vi "Create Log video.vi"(8 "error in (no error)":errorcluster, 11 "Acceleration Exceeded Log Folder":path=path "c:/logfiles") -> (0 "error out":errorcluster, 2 "AVI Refnum":T2)   [LabVIEW 2017]
uses:
  <vilib>/vision/Avi.llb/IMAQ AVI2 Refnum.ctl
  <vilib>/vision/Image Controls.llb/IMAQ Image.ctl
  <vilib>/userdefined/High Color/IMAQdx.ctl
  <vilib>/vision/driver/NI_Vision_Acquisition_Software.lvlib
panel:
  out "New Image":T1
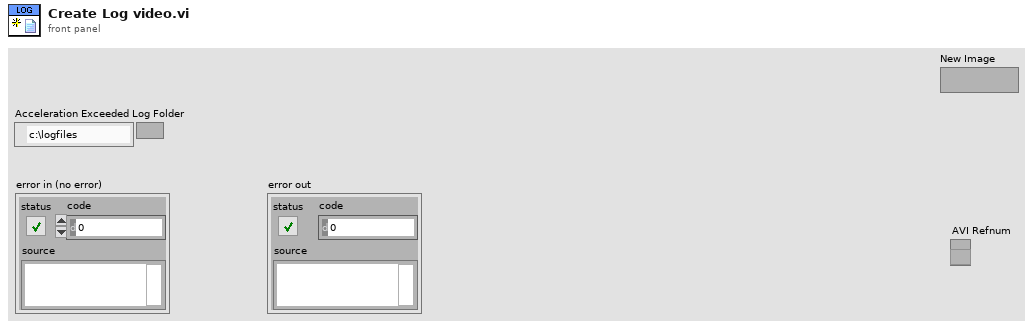
[diagram p1: front panel]
types:
  T1 = typedef "IMAQ Image.ctl" = refnum<image>
  T2 = typedef "IMAQ AVI2 Refnum.ctl" = refnum<k20>
  T3 = typedef "IMAQdx.ctl" = refnum<k21>
  T4 = typedef "Image Type" = u32
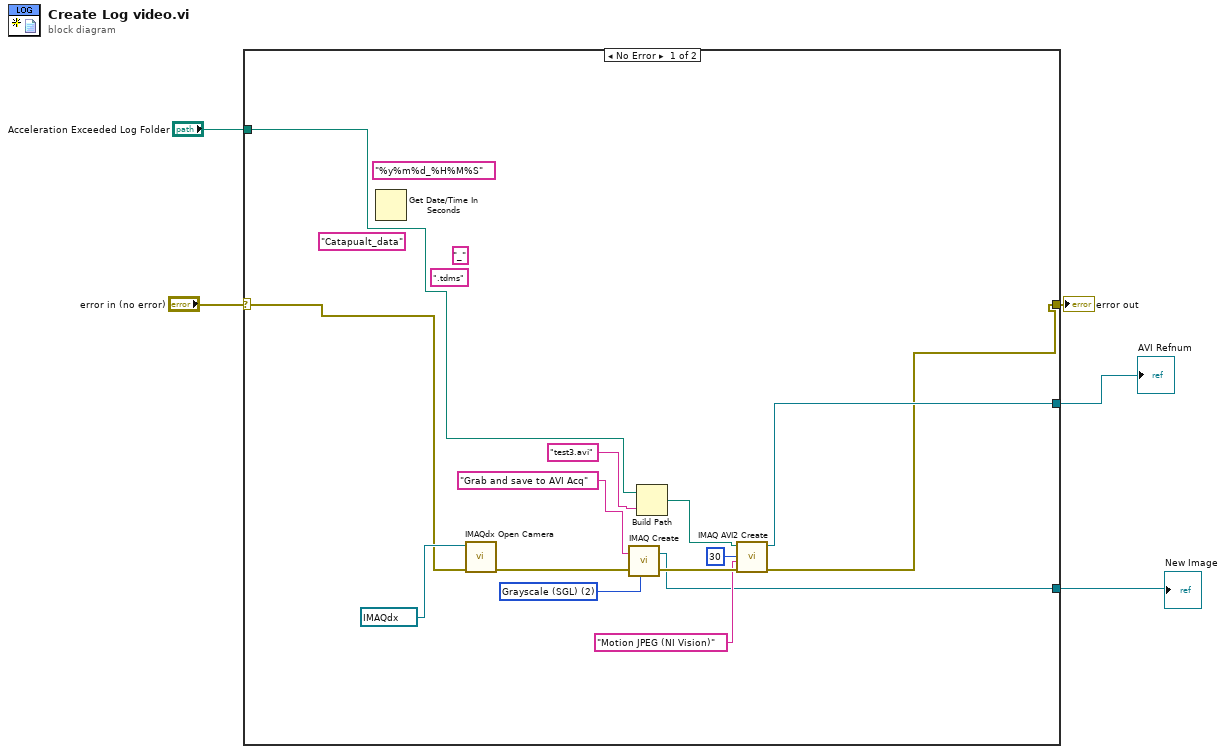
[diagram p0: block diagram]
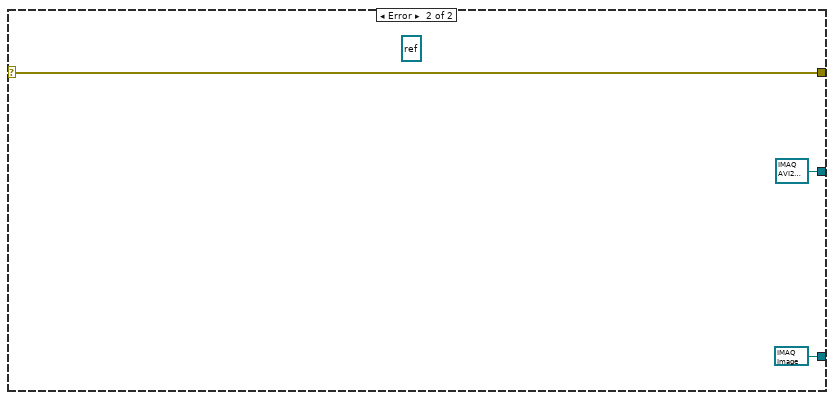
[diagram p2: hidden frame]
diagram:
  n1 = case shown="No Error" "error in (no error)" {
    selector: "error in (no error)" -> [w10 w22]
    tunnel: [w7 w22] -> w5
    tunnel: "Acceleration Exceeded Log Folder" -> [w8 _]
    tunnel: [w9 T2 refnum ("AVI Refnum")] -> w2
    tunnel: [w6 T1 refnum ("New Image")] -> w1
    frame No Error {
      w14 = T4 2 items=["Grayscale (U8)", "Grayscale (I16)", "Grayscale (SGL)", "Complex (CSG)", "RGB (U32)", "HSL (U32)", "RGB (U64)", "Grayscale (U16)"] ("Image Type")
      (unwired) "Catapualt_data" ("string")
      (unwired) "_" ("string")
      (unwired) ".tdms" ("string")
      (unwired) "%y%m%d_%H%M%S" ("time format string (%c)")
      n2 = Get Date/Time In Seconds() -> ()  [unwired: 1 out]
      n3 = call <vilib>:"IMAQdx Open Camera.vi"("error in"=w10, "Session In"=T3 "cam0") -> ("error out"=w18:errorcluster)  [unwired: 8 in, 1 out]
      n4 = call "IMAQ Create"("Image Name"="Grab and save to AVI Acq", "Image Type"=w14, "error in (no error)"=w18) -> ("New Image"=w6:T1, "error out"=w19:errorcluster)  [unwired: 2 in]
      n5 = Build Path(base path=w8, name or relative path="test3.avi") -> (appended path=w17:path)
      n6 = call "IMAQ AVI2 Create"("error in (no error)"=w19, "Codec"="Motion JPEG (NI Vision)", "Frames Per Second"=u32 30, "AVI Path"=w17) -> ("error out"=w7:errorcluster, "AVI Refnum"=w9:T2)  [unwired: 6 in]
    }
    frame Error {
      (unwired) refnum<k34> refnum ("tdms file out")
    }
  }
  "error out" <- w5
  "AVI Refnum" <- w2
  "New Image" <- w1
